vi "GetWarnings.vi"(1 "Deviceindex":i32) -> (0 "warningstext":string)   [LabVIEW 2011]
uses:
  MT Scan/SubVIs/hhlib.dll
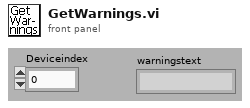
[diagram p1: front panel]
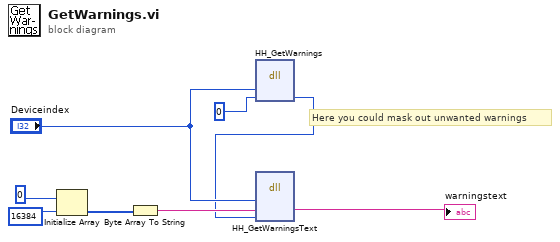
[diagram p0: block diagram]
diagram:
  # "Here you could mask out unwanted warnings"
  n1 = Initialize Array "Initialize Array"(u8 0, 16384) -> (w5:u8[])
  n2 = Byte Array To String(unsigned byte array=w5) -> (string=w4:string)
  n3 = dll-call lib="C:/Users/Core-FCS/Desktop/AbelFCS/MT Scan/SubVIs/hhlib.dll" fn="HH_GetWarnings"("devidx"="Deviceindex", "warnings"=0) -> ("warnings"=w1:i32)  [unwired: 5 in, 2 out]
  n4 = dll-call lib="C:/Users/Core-FCS/Desktop/AbelFCS/MT Scan/SubVIs/hhlib.dll" fn="HH_GetWarningsText"("devidx"="Deviceindex", "warningstext"=w4, "warnings"=w1) -> ("warningstext"=→"warningstext":string)  [unwired: 6 in, 2 out]
